vi "SwissSPAD Live_Globals.vi"() -> ()   [LabVIEW 2021]
panel:
  out "Abort":bool
  in  "Admin":bool
  in  "Settings Window Refnum":refnum<vi>
  in  "SwissSPAD Live Version":string
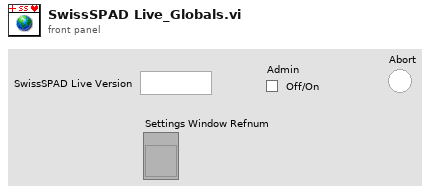
[diagram p1: front panel]
diagram:
